vi "Configure Modulation (Pulse).vi"(0 "VISA resource name":refnum<visa-resource-name>, 1 "Enable Pulse Modulation (T:Enable)":bool=TRUE, 2 "Pulse Modulation Source (1: Internal Free-Run)":u16(ring)=1 items=["Internal Square", "Internal Free-Run", "Internal Triggered", "Internal Adjustable Doublet", "Internal Doublet", "Internal Gated", "External Pulse", "Scalar"], 3 "Pulse Rate (400 Hz)":dbl=400.0, 5 "Pulse Delay1 (0 s)":dbl, 7 "Pulse Delay2 (0 s)":dbl, 9 "Pulse Period (4 us)":dbl=4e-06, 11 "error in (no error)":errorcluster, 12 "Pulse Width1 (1 us)":dbl=1e-06, 13 "Pulse Width2 (2 us)":dbl=2e-06, 14 "External Polarity (0: Normal)":u16(ring) items=["Normal", "Inverted"]) -> (4 "VISA resource name out":refnum<visa-resource-name>, 15 "error out":errorcluster)   [LabVIEW 2014, in "Agilent PSG MXG Series.lvlib"]
doc: "Configures pulse modulation.\n\n<B>Notes:</B>\n(1) This VI is <B>NOT</B> valid in E8247C.\n\n(2) For N5161A, N5162A, N5181A, N5182A, N5183A, this VI is valid only when the instrument installs <B>Option UNU</B> (Pulse modulation) and <B>Option UNW</B> (Narrow pulse modulation).\n\n(3) For N5171B, N5172B, N5181B, N5182B, this VI is valid only when the instrument installs <B>Option UNW</B> (Narrow pulse modulation).\n\n(4) For E8257D, E8267D, this VI is valid only when the instrument installs <B>Option UNU</B> or <B>Option UNW</B>."
uses:
  Agilent PSG MXG Series.lvlib
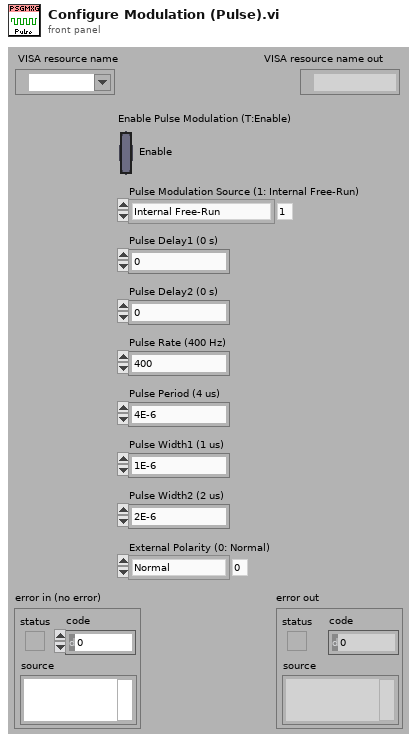
[diagram p1: front panel]
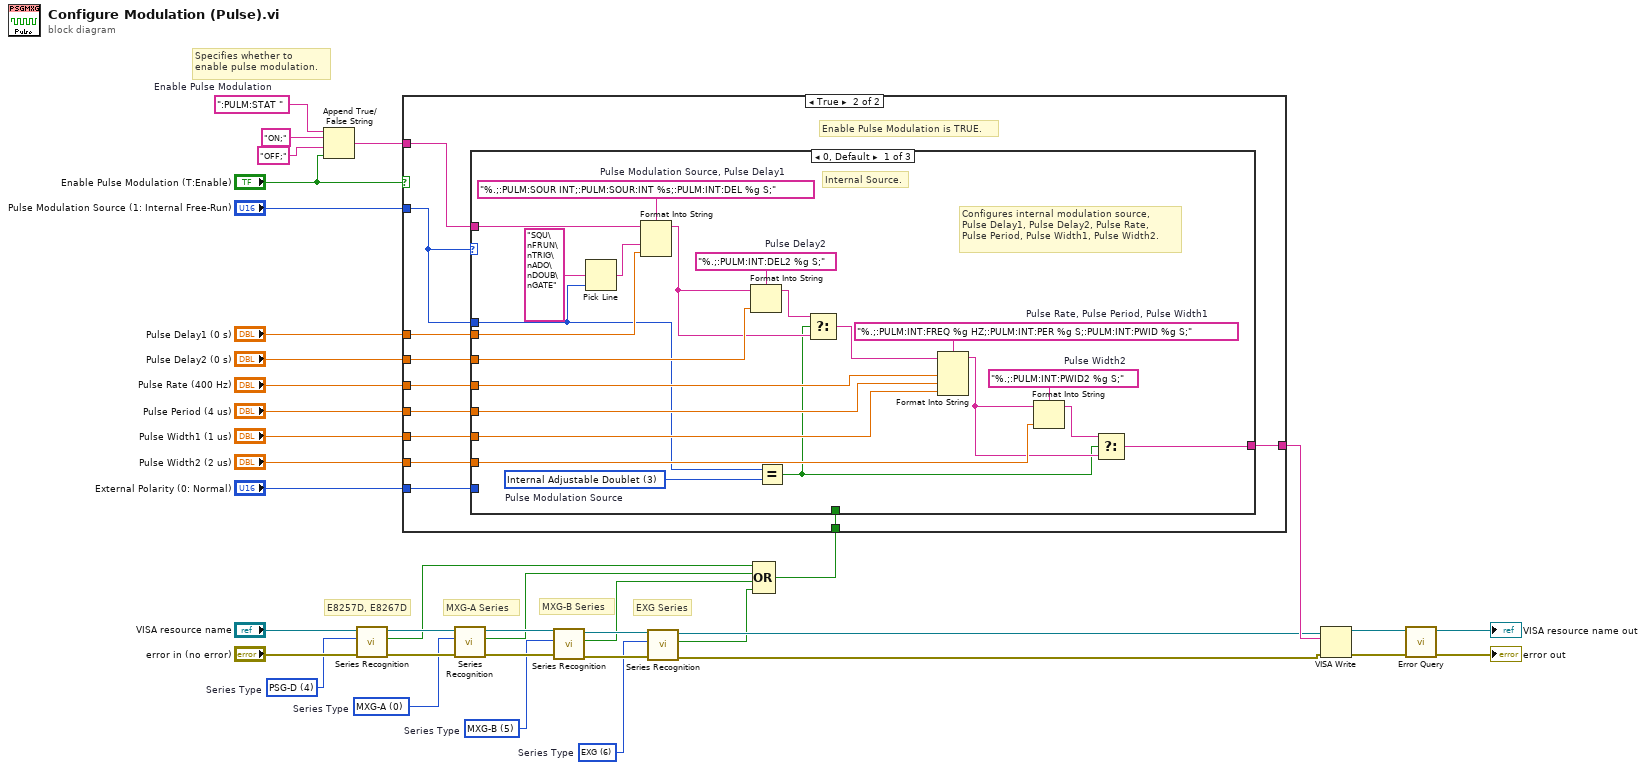
[diagram p0: block diagram]
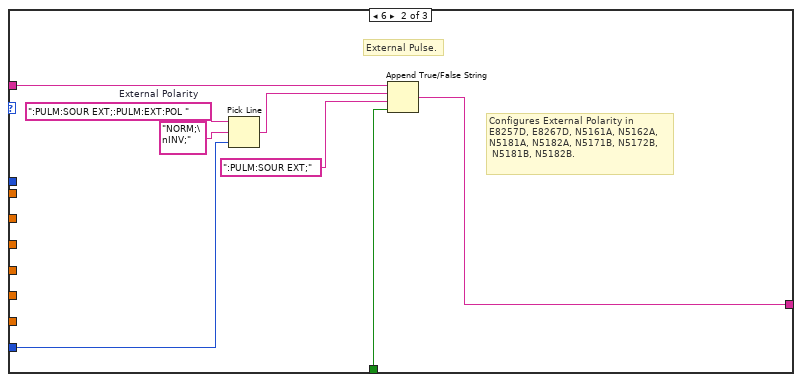
[diagram p3: hidden frame]
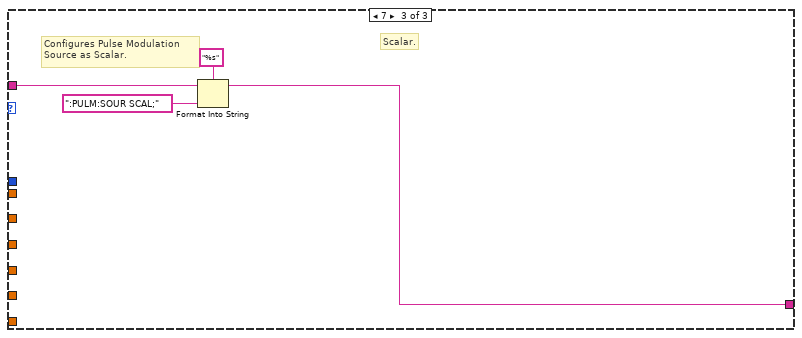
[diagram p4: hidden frame]
diagram:
  w6 = u16 6 items=["MXG-A", "PSG", "PSG-A", "PSG-C", "PSG-D", "MXG-B", "EXG"]  # Series Type
  w7 = u16 5 items=["MXG-A", "PSG", "PSG-A", "PSG-C", "PSG-D", "MXG-B", "EXG"]  # Series Type
  w14 = u16 0 items=["MXG-A", "PSG", "PSG-A", "PSG-C", "PSG-D", "MXG-B", "EXG"]  # Series Type
  w15 = u16 4 items=["MXG-A", "PSG", "PSG-A", "PSG-C", "PSG-D", "MXG-B", "EXG"]  # Series Type
  w37 = ":PULM:STAT "  # Enable Pulse Modulation
  # "EXG Series"
  # "MXG-B Series"
  # "Specifies whether to\nenable pulse modulation."
  # "E8257D, E8267D"
  # "MXG-A Series"
  n1 = Append True/False String(1:"Enable Pulse Modulation (T:Enable)", 2:"OFF;" ("false string"), 3:"ON;" ("true string"), 4:w37) -> (0:w32:string)
  n2 = call "Series Recognition.vi"("error in (no error)"="error in (no error)", "Series Type (0: MXG)"=w15, "VISA resource name"="VISA resource name") -> ("error out"=w20:errorcluster, "Is Series Correct"=w2:bool, "VISA resource name out"=w21:refnum<visa-resource-name>)  [unwired: 6 out]
  n3 = call "Series Recognition.vi"("error in (no error)"=w20, "Series Type (0: MXG)"=w14, "VISA resource name"=w21) -> ("error out"=w11:errorcluster, "Is Series Correct"=w3:bool, "VISA resource name out"=w13:refnum<visa-resource-name>)  [unwired: 6 out]
  n4 = call "Series Recognition.vi"("error in (no error)"=w11, "Series Type (0: MXG)"=w7, "VISA resource name"=w13) -> ("error out"=w10:errorcluster, "Is Series Correct"=w4:bool, "VISA resource name out"=w12:refnum<visa-resource-name>)  [unwired: 6 out]
  n5 = call "Series Recognition.vi"("error in (no error)"=w10, "Series Type (0: MXG)"=w6, "VISA resource name"=w12) -> ("error out"=w8:errorcluster, "Is Series Correct"=w5:bool, "VISA resource name out"=w9:refnum<visa-resource-name>)  [unwired: 6 out]
  n6 = Compound Arithmetic op=OR(w2, w3, w4, w5) -> (w1:bool)
  n7 = case shown="True" "Enable Pulse Modulation (T:Enable)" {
    tunnel: "Pulse Modulation Source (1: Internal Free-Run)" -> [_ w40]
    tunnel: w32 -> [w38 w49]
    tunnel: "Pulse Delay1 (0 s)" -> [_ w48]
    tunnel: "Pulse Delay2 (0 s)" -> [_ w47]
    tunnel: "Pulse Rate (400 Hz)" -> [_ w46]
    tunnel: "Pulse Period (4 us)" -> [_ w45]
    tunnel: "Pulse Width1 (1 us)" -> [_ w44]
    tunnel: "Pulse Width2 (2 us)" -> [_ w43]
    tunnel: "External Polarity (0: Normal)" -> [_ w42]
    tunnel: [w38 w41] -> w24
    tunnel: w1 -> [_ w39]
    frame False {
      # "Enable Pulse Modulation is FALSE."
    }
    frame True {
      # "Enable Pulse Modulation is TRUE."
      n8 = case shown="0, Default" w40 {
        tunnel: w40 -> [w51 _ _]
        tunnel: w49 -> [w67 w74 w83]
        tunnel: w48 -> [w66 _ _]
        tunnel: w47 -> [w65 _ _]
        tunnel: w46 -> [w60 _ _]
        tunnel: w45 -> [w59 _ _]
        tunnel: w44 -> [w57 _ _]
        tunnel: w43 -> [w56 _ _]
        tunnel: w42 -> [_ w77 _]
        tunnel: [w53 w73 w80] -> w41
        tunnel: w39 -> [_ w72 _]
        frame 0, Default {
          w52 = u16 3 items=["Internal Square", "Internal Free-Run", "Internal Triggered", "Internal Adjustable Doublet", "Internal Doublet", "Internal Gated", "External Pulse", "Scalar"]  # Pulse Modulation Source
          w58 = "%.;:PULM:INT:PWID2 %g S;"  # Pulse Width2
          w61 = "%.;:PULM:INT:FREQ %g HZ;:PULM:INT:PER %g S;:PULM:INT:PWID %g S;"  # Pulse Rate, Pulse Period, Pulse Width1
          w68 = "%.;:PULM:SOUR INT;:PULM:SOUR:INT %s;:PULM:INT:DEL %g S;"  # Pulse Modulation Source, Pulse Delay1
          w69 = "%.;:PULM:INT:DEL2 %g S;"  # Pulse Delay2
          # "Configures internal modulation source,\nPulse Delay1, Pulse Delay2, Pulse Rate,\nPulse Period, Pulse Width1, Pulse Width2."
          # "Internal Source."
          n9 = Pick Line(multi-line string="SQU\nFRUN\nTRIG\nADO\nDOUB\nGATE", line index=w51) -> (output string=w70:string)  [unwired: 1 out]
          n10 = Format Into String(format string=w68, initial string=w67, w70, w66) -> (resulting string=w63:string)  [unwired: 1 in, 1 out]
          n11 = Format Into String(format string=w69, initial string=w63, w65) -> (resulting string=w64:string)  [unwired: 1 in, 1 out]
          n12 = Equal?(x=w51, y=w52) -> (x = y?=w50:bool)
          n13 = Select(t=w64, s=w50, f=w63) -> (s? t:f=w62:string)
          n14 = Format Into String(format string=w61, initial string=w62, w60, w59, w57) -> (resulting string=w54:string)  [unwired: 1 in, 1 out]
          n15 = Format Into String(format string=w58, initial string=w54, w56) -> (resulting string=w55:string)  [unwired: 1 in, 1 out]
          n16 = Select(t=w55, s=w50, f=w54) -> (s? t:f=w53:string)
        }
        frame 6 {
          w79 = ":PULM:SOUR EXT;:PULM:EXT:POL "  # External Polarity
          # "Configures External Polarity in\nE8257D, E8267D, N5161A, N5162A, \nN5181A, N5182A, N5171B, N5172B,\n N5181B, N5182B."
          # "External Pulse."
          n17 = Pick Line(string ("")=w79, multi-line string="NORM;\nINV;", line index=w77) -> (output string=w76:string)
          n18 = Append True/False String(1:w72, 2:":PULM:SOUR EXT;" ("false string"), 3:w76, 4:w74) -> (0:w73:string)
        }
        frame 7 {
          # "Configures Pulse Modulation\nSource as Scalar."
          # "Scalar."
          n19 = Format Into String(format string="%s", initial string=w83, ":PULM:SOUR SCAL;" ("true string")) -> (resulting string=w80:string)  [unwired: 1 in, 1 out]
        }
      }
    }
  }
  n20 = VISA Write(VISA resource name=w9, write buffer=w24, error in (no error)=w8) -> (VISA resource name out=w23:refnum<visa-resource-name>, error out=w22:errorcluster)  [unwired: 1 out]
  n21 = call "Error Query.vi"("error in (no error)"=w22, "VISA resource name"=w23) -> ("error out"=→"error out":errorcluster, "VISA resource name out"=→"VISA resource name out":refnum<visa-resource-name>)  [unwired: 8 out]
